vi "run.vi"(8 "error in (no error)":errorcluster, 11 "DL090623TwoDAnalyser in":refnum<class "AnalyserDL090623TwoD.lvclass">) -> (0 "error out":errorcluster, 3 "DL090623TwoDAnalyser out":refnum<class "AnalyserDL090623TwoD.lvclass">)   [LabVIEW 2010, in "AnalyserDL090623TwoD.lvclass"]
uses:
  AnalyserDL090623TwoD.lvclass
  AnalyserDL090623TwoD.lvclass/AnalyserDL090623TwoD.ctl
  AnalyserDL090624Scaffold/AnalyserDL090624Scaffold/AnalyserDL090624Scaffold.lvclass
  <vilib>/vision/Image Controls.llb/IMAQ Image.ctl
  common/classes/Image/Image/Image.lvclass
  Display/GenericDisplay/GenericDisplay/GenericDisplay.lvclass
  common/classes/ErrorController/ErrorController/class_data.vi
  GenericAnalyser/GenericAnalyser/GenericAnalyser.lvclass
  common/classes/ErrorController/ErrorController/ErrorController.lvclass
panel:
  in  "obtain-background button":bool
  in  "get displayed image button":bool
  out "event handling loop error":errorcluster
  out "finished?":bool
  in  "Tab Control":enum32{"0", "1", "2", "3", "4"}(tab)
  in  "segment button":bool
  in  "load-reference-image button":bool
  out "reference image":T1(plugin-control)
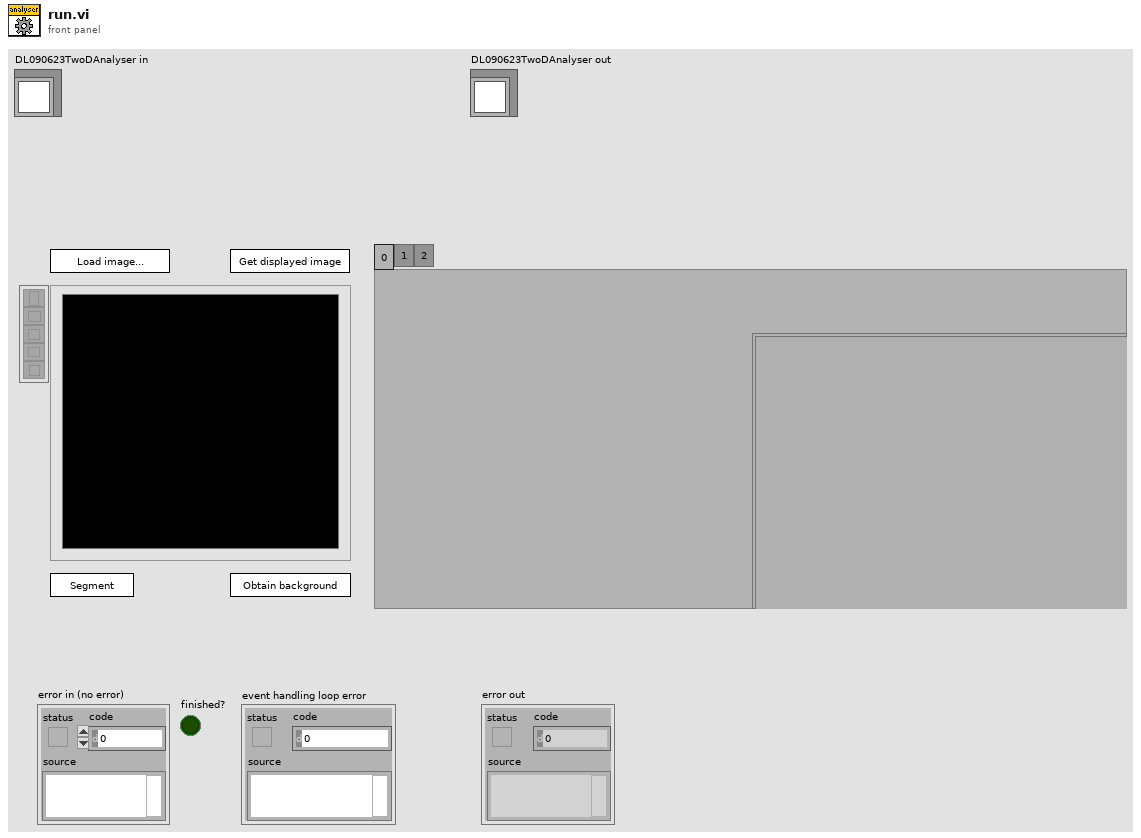
[diagram p1: front panel]
types:
  T1 = typedef "IMAQ Image.ctl" = refnum<image>
  T2 = cluster{"Global Rectangle":i32[], "Contours":cluster{"Contour Type":u32, "ROI Type":u32, "Points":i32[]}[]}
  T3 = typedef "ROI Descriptor" = cluster{"Global Rectangle":i32[], "Contours":cluster{"ID":enum32{"External", "Internal"}, "Type":u32, "Coordinates":i32[]}[]}
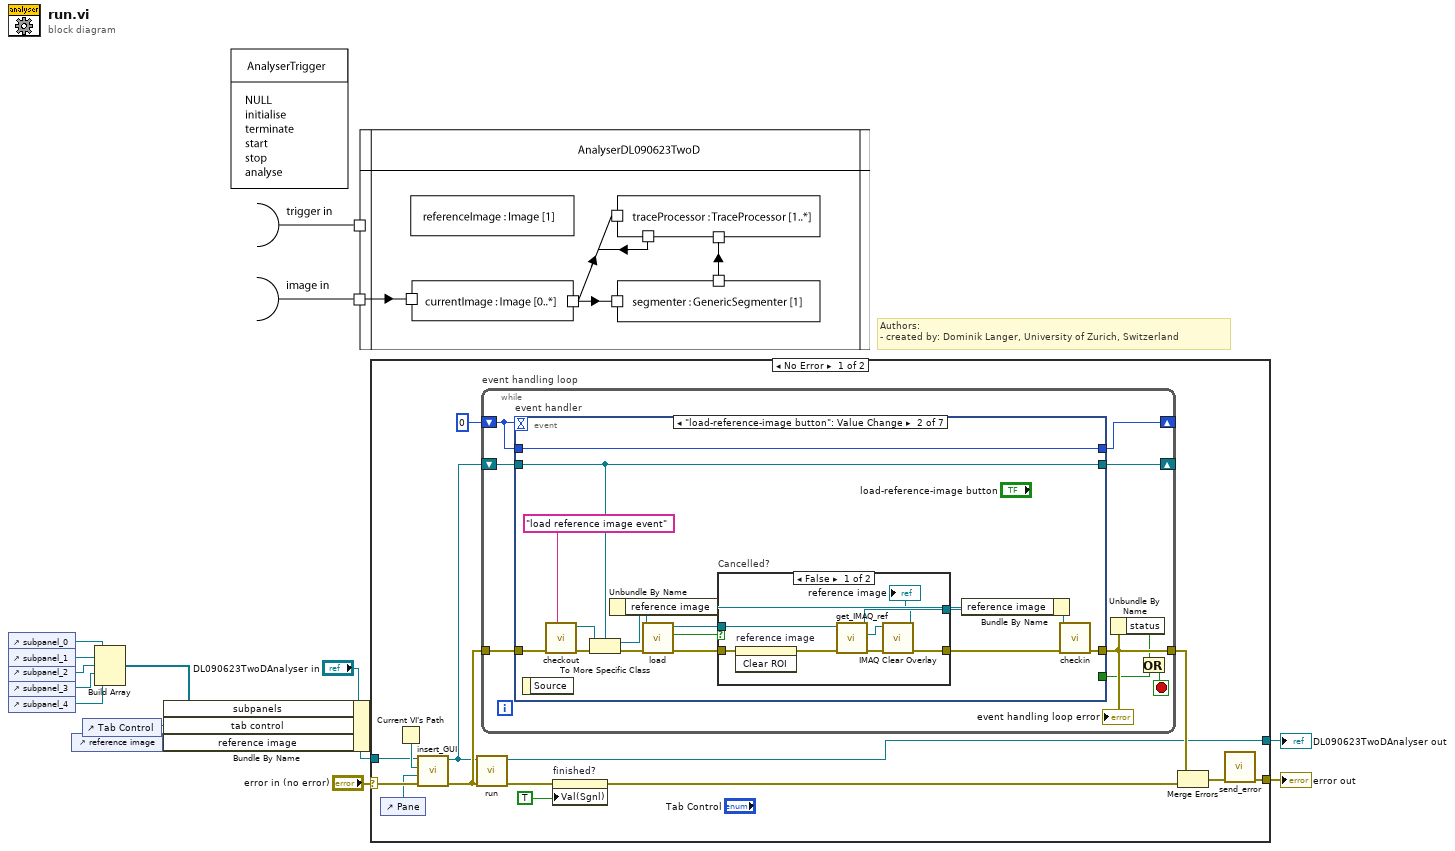
[diagram p0: block diagram]
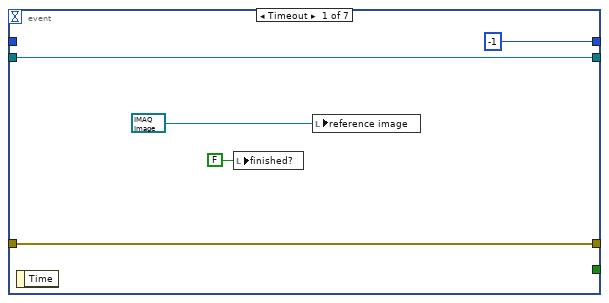
[diagram p2: hidden frame]
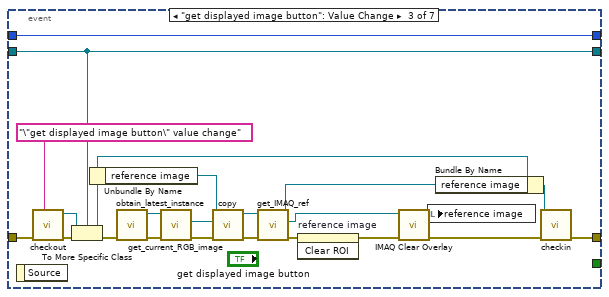
[diagram p4: hidden frame]
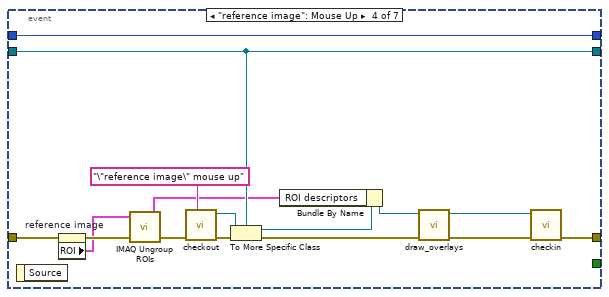
[diagram p5: hidden frame]
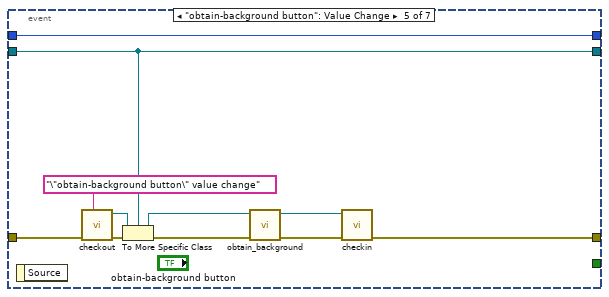
[diagram p6: hidden frame]
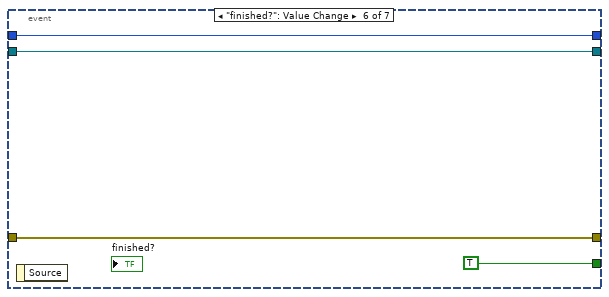
[diagram p7: hidden frame]
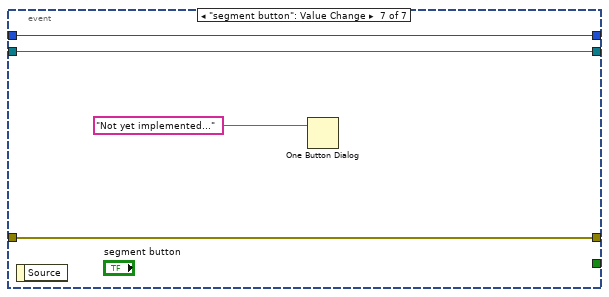
[diagram p8: hidden frame]
diagram:
  # "Authors: \n- created by: Dominik Langer, University of Zurich, Switzerland"
  n1 = control-ref of="subpanel_0"() -> (w8:refnum<vi>)
  n2 = control-ref of="subpanel_1"() -> (w7:refnum<vi>)
  n3 = control-ref of="subpanel_2"() -> (w6:refnum<vi>)
  n4 = control-ref of="subpanel_3"() -> (w4:refnum<vi>)
  n5 = control-ref of="subpanel_4"() -> (w3:refnum<vi>)
  n6 = control-ref of="reference image"() -> (w1:refnum<vi>)
  n7 = control-ref of="Tab Control"() -> (w2:refnum<vi>)
  n8 = Build Array(w8, w7, w6, w4, w3) -> (w5:refnum<vi>[])
  n9 = Bundle By Name(cluster="DL090623TwoDAnalyser in", "subpanels"=w5, "tab control"=w2, "reference image"=w1) -> (w9:refnum<class "AnalyserDL090623TwoD.lvclass">)
  n10 = case shown="No Error" "error in (no error)" {
    selector: "error in (no error)" -> [w17 w127]
    tunnel: [w14 w127] -> w12
    tunnel: [w25 w126] -> w11
    tunnel: w9 -> [w18 w126]
    frame No Error {
      n11 = control-ref of="Pane"() -> (w16:refnum<vi>)
      n12 = Current VI's Path() -> (path=w21:path)
      n13 = call-dynamic "insert_GUI.vi"("error in (no error)"=w17, "Pane"=w16, "VI path"=w21, "GenericComponent in"=w18) -> ("error out"=w20:errorcluster, "GenericComponent out"=w19:refnum<class "AnalyserDL090623TwoD.lvclass">)  [unwired: 6 in]
      n14 = call-parent "run.vi"("error in (no error)"=w20, "DL090624AnalyserScaffold in"=w19) -> ("error out"=w23:errorcluster, "DL090624AnalyserScaffold out"=w25:refnum<class "AnalyserDL090623TwoD.lvclass">)  [unwired: 8 out]
      n15 = while "event handling loop" {
        shift-right: [w35] -> _
        shift-left: 0 -> [w36]
        shift-right: [w33] -> _
        shift-left: w19 -> [w34]
        tunnel: w20 -> [w32]
        tunnel: [w31] -> w26
        stop <- w30 stop-if-true
        n16 = event "event handler" shown="[1] \"load-reference-image button\": Value Change" {
          selector: _ -> [_ _ _ _ _ _ _]
          dyn-events: _ -> [_ _ _ _ _ _ _]
          timeout: w36 -> [_ _ _ _ _ _ _]
          tunnel: [-1 w57 w90 w106 w117 w121 w125] -> w35
          tunnel: w36 -> [_ w57 w90 w106 w117 w121 w125]
          tunnel: [w40 w50 w72 w104 w113 w120 w124] -> w33
          tunnel: w34 -> [w40 w50 w72 w104 w113 w120 w124]
          tunnel: [w39 w51 w74 w95 w114 w119 w123] -> w31
          tunnel: w32 -> [w39 w44 w79 w105 w115 w119 w123]
          tunnel: [_ _ _ _ _ TRUE _] -> w29
          event Timeout {
            n17 = event-data() -> ()  [unwired: 2 out]
            n18 = local write "finished?"(FALSE ("finished?")) -> ()
            n19 = local write "reference image"(T1 refnum ("reference image")) -> ()
          }
          event "load-reference-image button": Value Change {
            n20 = event-data() -> ()  [unwired: 2 out]
            n21 = call "checkout.vi"("locked by?"="load reference image event", "error in (no error)"=w44) -> ("error out"=w55:errorcluster, "GeneralAnalyser out"=w53:refnum<class "GenericAnalyser.lvclass">)  [unwired: 8 in]
            n22 = To More Specific Class(target class=w50, reference=w53, error in=w55) -> (specific class reference=w49:refnum<class "AnalyserDL090623TwoD.lvclass">, error out=w54:errorcluster)
            n23 = Unbundle By Name(w49) -> ("reference image"=w52:refnum<class "Image.lvclass">)
            n24 = call-dynamic "load.vi"("error in (no error)"=w54, "Image in"=w52) -> ("error out"=w43:errorcluster, "cancelled?"=w42:bool, "Image out"=w56:refnum<class "Image.lvclass">)  [unwired: 2 in, 5 out]
            n25 = case "Cancelled?" shown="False" w42 {
              tunnel: w56 -> [w65 w66]
              tunnel: [w64 w66] -> w48
              tunnel: [w62 w67] -> w45
              tunnel: w43 -> [w59 w67]
              frame False {
                n26 = invoke on="reference image" class="ImageControl" method="Clear ROI"(error in=w59) -> (error out=w58:errorcluster)  [unwired: 2 in, 2 out]
                n27 = call-dynamic "get_IMAQ_ref.vi"("error in (no error)"=w58, "Image.lvclass in"=w65) -> ("error out"=w63:errorcluster, "Image"=w61:T1, "Image.lvclass out"=w64:refnum<class "Image.lvclass">)  [unwired: 7 out]
                n28 = call "IMAQ Clear Overlay"("error in (no error)"=w63, "Image"=w61) -> ("error out"=w62:errorcluster, "Image Out"=→"reference image":T1)  [unwired: 1 in, 7 out]
              }
              frame True {
              }
            }
            n29 = Bundle By Name(cluster=w49, "reference image"=w48) -> (w47:refnum<class "AnalyserDL090623TwoD.lvclass">)
            n30 = call-dynamic "checkin.vi"("error in (no error)"=w45, "GeneralAnalyser in"=w47) -> ("error out"=w51:errorcluster)  [unwired: 8 in, 1 out]
          }
          event "get displayed image button": Value Change {
            n31 = event-data() -> ()  [unwired: 2 out]
            n32 = call "checkout.vi"("locked by?"="\"get displayed image button\" value change", "error in (no error)"=w79) -> ("error out"=w78:errorcluster, "GeneralAnalyser out"=w76:refnum<class "GenericAnalyser.lvclass">)  [unwired: 8 in]
            n33 = To More Specific Class(target class=w72, reference=w76, error in=w78) -> (specific class reference=w71:refnum<class "AnalyserDL090623TwoD.lvclass">, error out=w77:errorcluster)
            n34 = Unbundle By Name(w71) -> ("reference image"=w86:refnum<class "Image.lvclass">)
            n35 = call "obtain_latest_instance.vi"("error in (no error)"=w77) -> ("error out"=w89:errorcluster, "GenericDisplay out"=w88:refnum<class "GenericDisplay.lvclass">)  [unwired: 1 in, 8 out]
            n36 = call-dynamic "get_current_RGB_image.vi"("error in (no error)"=w89, "GenericDisplay in"=w88) -> ("error out"=w85:errorcluster, "RGB image"=w84:refnum<class "Image.lvclass">)  [unwired: 8 out]
            n37 = call "copy.vi"("error in (no error)"=w85, "image to copy (source)"=w84, "Image in (target)"=w86) -> ("error out"=w83:errorcluster, "Image out"=w82:refnum<class "Image.lvclass">)  [unwired: 7 out]
            n38 = call-dynamic "get_IMAQ_ref.vi"("error in (no error)"=w83, "Image.lvclass in"=w82) -> ("error out"=w70:errorcluster, "Image"=w81:T1, "Image.lvclass out"=w80:refnum<class "Image.lvclass">)  [unwired: 7 out]
            n39 = invoke on="reference image" class="ImageControl" method="Clear ROI"(error in=w70) -> (error out=w69:errorcluster)  [unwired: 2 in, 2 out]
            n40 = call "IMAQ Clear Overlay"("error in (no error)"=w69, "Image"=w81) -> ("error out"=w68:errorcluster, "Image Out"=w87:T1)  [unwired: 1 in, 7 out]
            n41 = local write "reference image"(w87) -> ()
            n42 = Bundle By Name(cluster=w71, "reference image"=w80) -> (w73:refnum<class "AnalyserDL090623TwoD.lvclass">)
            n43 = call-dynamic "checkin.vi"("error in (no error)"=w68, "GeneralAnalyser in"=w73) -> ("error out"=w74:errorcluster)  [unwired: 8 in, 1 out]
          }
          event "reference image": Mouse Up {
            n44 = event-data() -> ()  [unwired: 2 out]
            n45 = property on="reference image" class="ImageControl"(error in=w105) -> (error out=w100:errorcluster, "ROI"=w98:T2)  [unwired: 1 in, 1 out]
            n46 = call "IMAQ Ungroup ROIs"("error in (no error)"=w100, "ROI Descriptor"=w98) -> ("error out"=w99:errorcluster, "ROI Descriptors out"=w96:T3[])  [unwired: 2 out]
            n47 = call "checkout.vi"("locked by?"="\"reference image\" mouse up", "error in (no error)"=w99) -> ("error out"=w103:errorcluster, "GeneralAnalyser out"=w101:refnum<class "GenericAnalyser.lvclass">)  [unwired: 8 in]
            n48 = To More Specific Class(target class=w104, reference=w101, error in=w103) -> (specific class reference=w97:refnum<class "AnalyserDL090623TwoD.lvclass">, error out=w94:errorcluster)
            n49 = Bundle By Name(cluster=w97, "ROI descriptors"=w96) -> (w93:refnum<class "AnalyserDL090623TwoD.lvclass">)
            n50 = call-dynamic "draw_overlays.vi"("error in (no error)"=w94, "DL090623TwoDAnalyser in"=w93) -> ("error out"=w92:errorcluster, "DL090623TwoDAnalyser out"=w91:refnum<class "AnalyserDL090623TwoD.lvclass">)  [unwired: 8 out]
            n51 = call-dynamic "checkin.vi"("error in (no error)"=w92, "GeneralAnalyser in"=w91) -> ("error out"=w95:errorcluster)  [unwired: 8 in, 1 out]
          }
          event "obtain-background button": Value Change {
            n52 = event-data() -> ()  [unwired: 2 out]
            n53 = call "checkout.vi"("locked by?"="\"obtain-background button\" value change", "error in (no error)"=w115) -> ("error out"=w116:errorcluster, "GeneralAnalyser out"=w112:refnum<class "GenericAnalyser.lvclass">)  [unwired: 8 in]
            n54 = To More Specific Class(target class=w113, reference=w112, error in=w116) -> (specific class reference=w108:refnum<class "AnalyserDL090623TwoD.lvclass">, error out=w110:errorcluster)
            n55 = call-dynamic "obtain_background.vi"("error in (no error)"=w110, "DL090623TwoDAnalyser in"=w108) -> ("error out"=w109:errorcluster, "DL090623TwoDAnalyser out"=w107:refnum<class "AnalyserDL090623TwoD.lvclass">)  [unwired: 8 out]
            n56 = call-dynamic "checkin.vi"("error in (no error)"=w109, "GeneralAnalyser in"=w107) -> ("error out"=w114:errorcluster)  [unwired: 8 in, 1 out]
          }
          event "finished?": Value Change {
            n57 = event-data() -> ()  [unwired: 2 out]
          }
          event "segment button": Value Change {
            n58 = event-data() -> ()  [unwired: 2 out]
            n59 = One Button Dialog(message="Not yet implemented...") -> ()  [unwired: 2 out]
          }
        }
        "event handling loop error" <- w31
        n60 = Unbundle By Name(w31) -> ("status"=w28:bool)
        n61 = Or(x=w28, y=w29) -> (x .or. y?=w30:bool)
      }
      n62 = property on="finished?" class="Bool (strict)"(error in=w23, "Val(Sgnl)"=TRUE) -> (error out=w22:errorcluster)  [unwired: 1 in, 1 out]
      n63 = Merge Errors(w26, w22) -> (w15:errorcluster)
      n64 = call "send_error.vi"("error in (no error)"=w15) -> ("error out"=w14:errorcluster)  [unwired: 10 in]
    }
    frame Error {
    }
  }
  "error out" <- w12
  "DL090623TwoDAnalyser out" <- w11
